vi "Measurement UI.vi"() -> ()   [LabVIEW 2025, in "CAN-LIN Frame Generator UI.lvlib"]
uses:
  CAN-LIN Frame Generator UI.lvlib
panel:
  in  "DUT Pin":string(combo) caption="Pin name"
  in  "CAN Interface":string
  in  "Termination CAN":bool
  in  "PAYLOAD":u32[](array[numeric])=[0, 1, 2, 3, 4, 5, 6, 7] format="%2x"
  in  "TYPE":u32(ring) items=["CAN Data"=0, "CAN Remote"=1, "CAN Bus Error"=2, "CAN 2.0 Data"=8, "CAN FD Data"=16, "CAN FD+BRS Data"=24, "J1939 Data"=192, "Delay"=224, "Log Trigger"=225, "Start Trigger"=226]
  in  "IDENTIFIER":u32=1034 format="%x"
  in  "IO Mode":enum32{"CAN", "CAN FD", "CAN FD + BRS"}(ring)
  in  "FD ISO Mode":enum32{"ISO", "Legacy ISO", "Non-ISO"}(ring)=enum."Non-ISO"
  in  "Baudrate":u32=125000 format="%x"
  in  "FD Baudrate":u32 format="%x"
  in  "INTERFACE NAME CAN":refnum<k21>="CAN1"
  # "CAN Settings"
  # "CAN Frame"
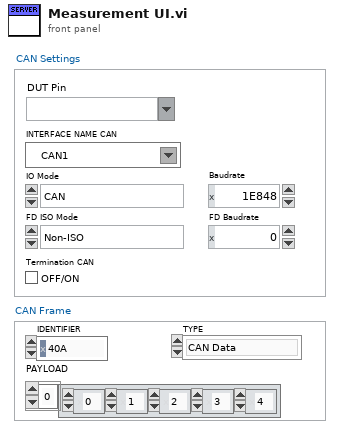
[diagram p1: front panel]
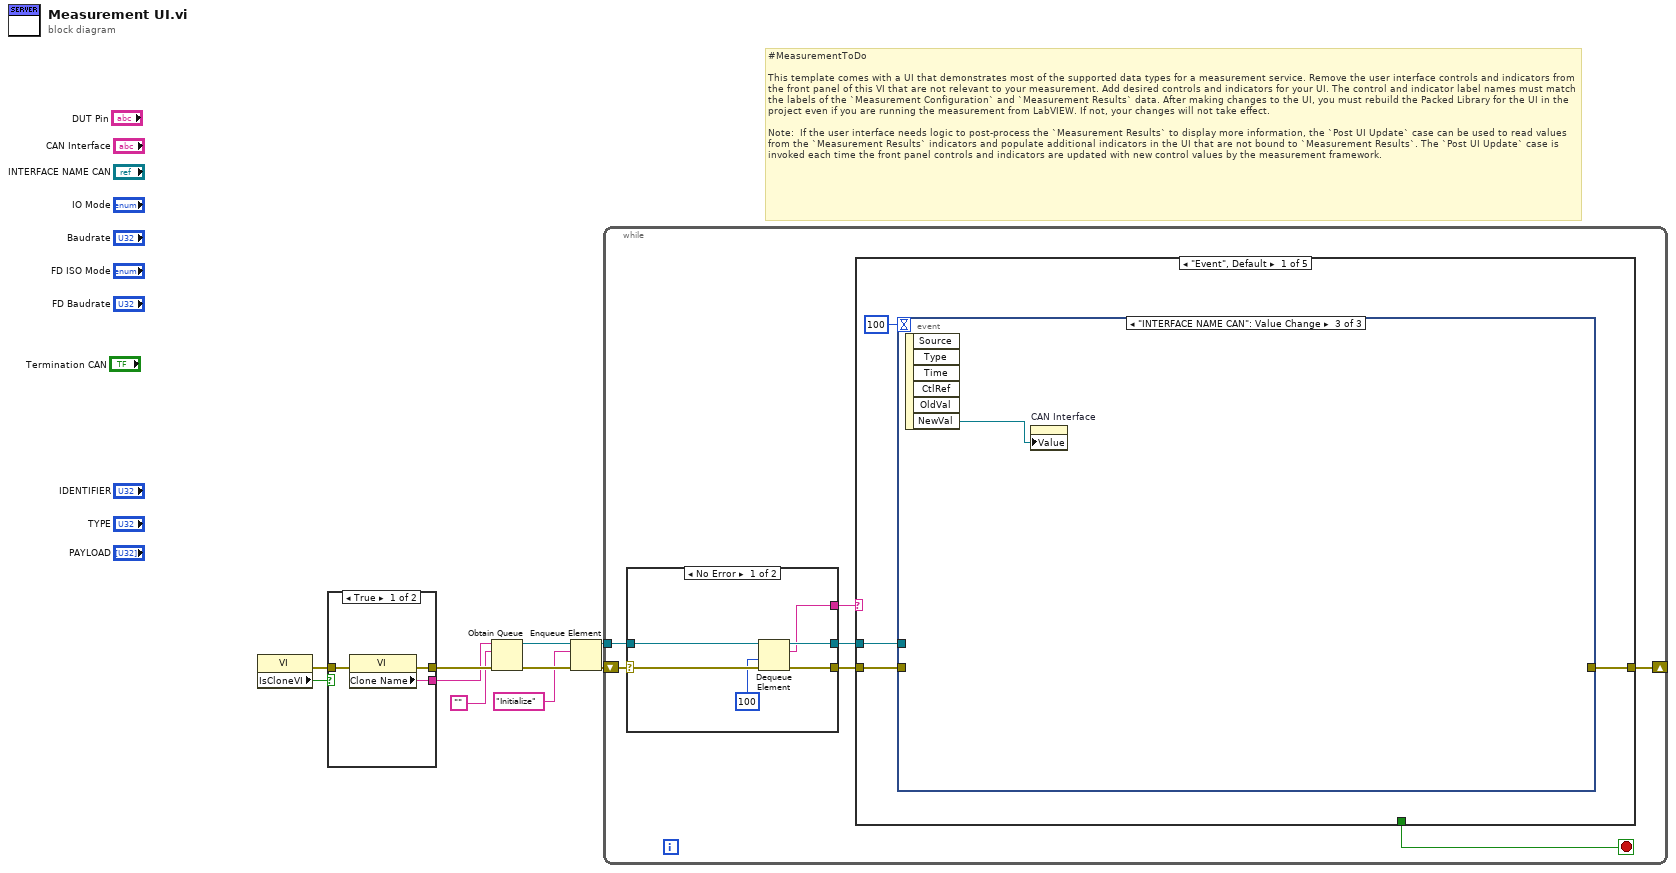
[diagram p0: block diagram]
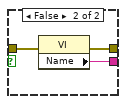
[diagram p2: hidden frame]
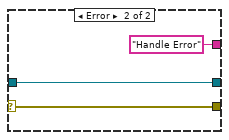
[diagram p3: hidden frame]
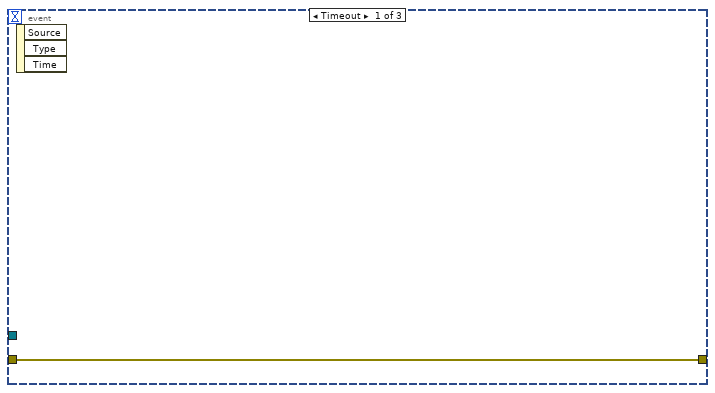
[diagram p4: hidden frame]
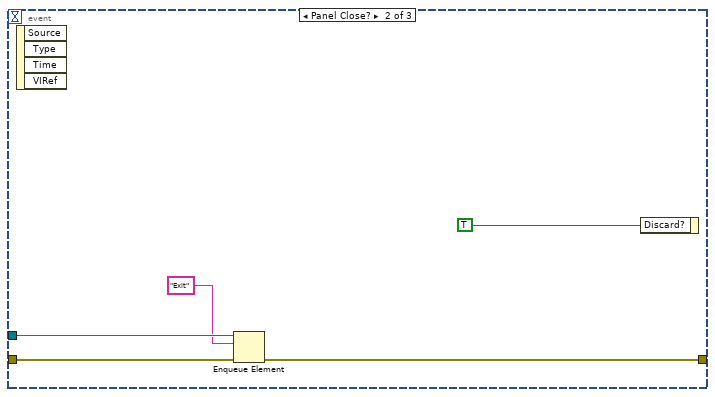
[diagram p5: hidden frame]
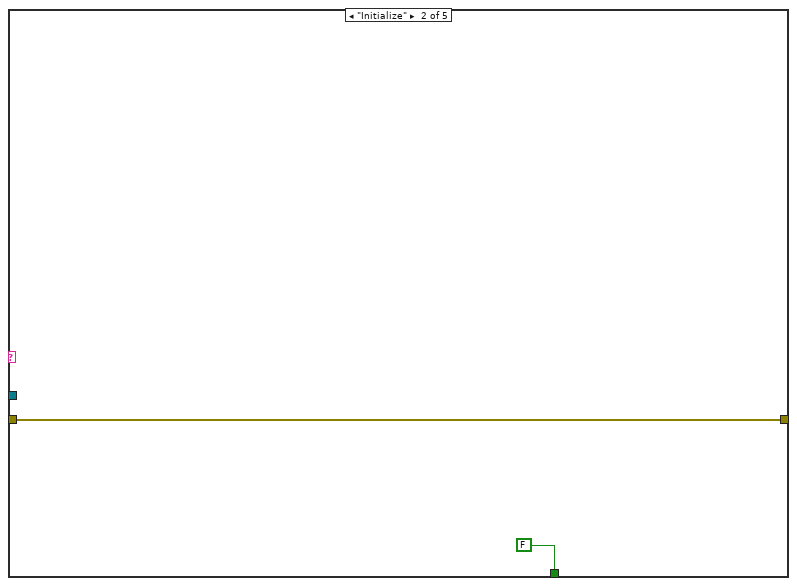
[diagram p6: hidden frame]
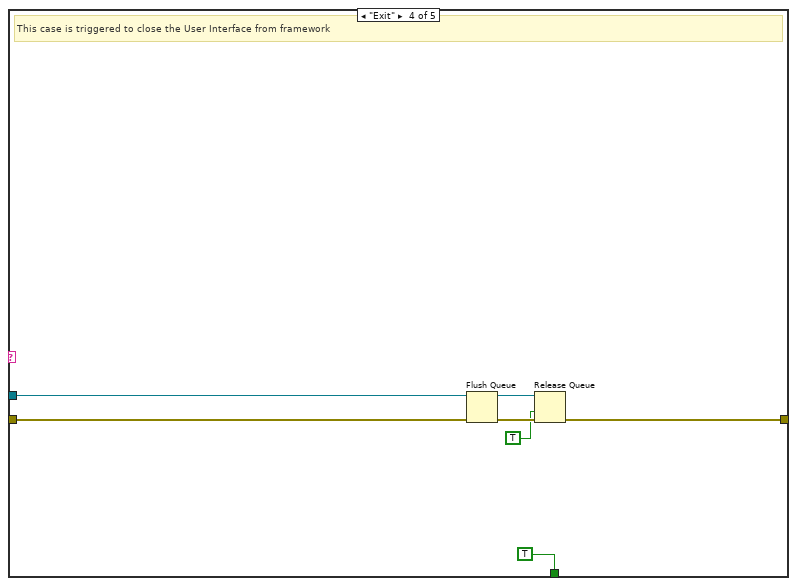
[diagram p8: hidden frame]
diagram:
  # "#MeasurementToDo  \n\nThis template comes with a UI that demonstrates most of the supported data types for a measurement service. Remove the user interface controls and indicators from the front panel of this VI that are not relevant to your measurement. Add desired controls and indicators for your UI. The control and indicator label names must match the labels of the `Measurement Configuration` and `Measurement Results` data. After making changes to the UI, you must rebuild the Packed Library for the UI in the project even if you are running the measurement from LabVIEW. If not, your changes will not take effect.\n\nNote:  If the user interface needs logic to post-process the `Measurement Results` to display more information, the `Post UI Update` case can be used to read values from the `Measurement Results` indicators and populate additional indicators in the UI that are not bound to `Measurement Results`. The `Post UI Update` case is invoked each time the front panel controls and indicators are updated with new control values by the measurement framework."
  n1 = property class="VI"() -> (error out=w1:errorcluster, "IsCloneVI"=w2:bool)  [unwired: 2 in, 1 out]
  n2 = case shown="True" w2 {
    tunnel: [w13 w16] -> w10
    tunnel: [w12 w15] -> w9
    tunnel: w1 -> [w11 w14]
    frame True {
      n3 = property class="VI"(error in=w11) -> (error out=w13:errorcluster, "Clone Name"=w12:string)  [unwired: 1 in, 1 out]
    }
    frame False {
      n4 = property class="VI"(error in=w14) -> (error out=w16:errorcluster, "Name"=w15:string)  [unwired: 1 in, 1 out]
    }
  }
  n5 = Obtain Queue(name (unnamed)=w9, element data type="", error in (no error)=w10) -> (queue out=w6:refnum<queue>, error out=w8:errorcluster)  [unwired: 2 in, 1 out]
  n6 = Enqueue Element(queue=w6, element="Initialize", error in (no error)=w8) -> (queue out=w5:refnum<queue>, error out=w7:errorcluster)  [unwired: 1 in, 1 out]
  n7 = while {
    shift-right: [w18] -> _
    shift-left: w7 -> [w23]
    tunnel: w5 -> [w21]
    stop <- w17 stop-if-true
    n8 = case shown="No Error" w23 {
      selector: w23 -> [w29 w32]
      tunnel: [w28 w32] -> w22
      tunnel: w21 -> [w27 w31]
      tunnel: [w26 w31] -> w20
      tunnel: [w25 "Handle Error"] -> w19
      frame No Error {
        n9 = Dequeue Element(queue=w27, timeout in ms (-1)=100, error in (no error)=w29) -> (queue out=w26:refnum<queue>, element=w25:string, error out=w28:errorcluster)  [unwired: 1 out]
      }
      frame Error {
      }
    }
    n10 = case shown="\"Event\", Default" w19 {
      tunnel: w22 -> [w35 w45 w46 w53 w54]
      tunnel: w20 -> [w33 _ _ w51 _]
      tunnel: [w36 w45 w46 w48 w54] -> w18
      tunnel: [_ FALSE _ TRUE _] -> w17
      frame "Event", Default {
        n11 = event shown="[2] \"INTERFACE NAME CAN\": Value Change" {
          selector: _ -> [_ _ _]
          dyn-events: _ -> [_ _ _]
          timeout: 100 -> [_ _ _]
          tunnel: [w37 w40 _] -> w36
          tunnel: w35 -> [w37 w41 _]
          tunnel: w33 -> [_ w39 _]
          event Timeout {
            n12 = event-data() -> ()  [unwired: 1 in, 3 out]
          }
          event Panel Close? {
            n13 = event-data() -> ()  [unwired: 1 in, 4 out]
            n14 = Enqueue Element(queue=w39, element="Exit", error in (no error)=w41) -> (error out=w40:errorcluster)  [unwired: 1 in, 2 out]
            n15 = event-data("Discard?"=TRUE) -> ()  [unwired: 1 in, 1 out]
          }
          event "INTERFACE NAME CAN": Value Change {
            n16 = event-data() -> ("NewVal"=w43:refnum<k21>)  [unwired: 1 in, 5 out]
            n17 = property on="CAN Interface" class="Str"("Value"=w43) -> ()  [unwired: 2 in, 2 out]
          }
        }
      }
      frame "Initialize" {
      }
      frame "Post UI Update" {
        # "This case will be triggered, after framework updates the User interface with result values."
      }
      frame "Exit" {
        # "This case is triggered to close the User Interface from framework"
        n18 = Flush Queue(queue=w51, error in (no error)=w53) -> (queue out=w50:refnum<queue>, error out=w49:errorcluster)  [unwired: 1 out]
        n19 = Release Queue(queue=w50, force destroy? (F)=TRUE, error in (no error)=w49) -> (error out=w48:errorcluster)  [unwired: 2 out]
      }
      frame "Handle Error" {
      }
    }
  }
